vi "Ethernet Packet Counter for Testing.vi"() -> ()   [LabVIEW 2025]
uses:
  <vilib>/xnet/xnet.llb/XNET Frame Type Ethernet.ctl
  <vilib>/xnet/xnet.llb/XNET Create Session (Frame Output Stream).vi
  <vilib>/xnet/xnet.llb/XNET Write (Frame Ethernet).vi
  Automotive Ethernet Bus Monitor/Automotive Ethernet Bus Monitor.lvclass
panel:
  out "error out":errorcluster
  in  "destination MAC address":cluster{u8, u8, u8, u8, u8, u8}={255, 255, 255, 255, 255, 255} {"?" format="%.0x"; "?" format="%.0x"; "?" format="%.0x"; "?" format="%.0x"; "?" format="%.0x"; "?" format="%.0x"}
  in  "Has VLAN Tag 2":bool=TRUE
  in  "VID 2":u16=2
  in  "priority":u8=3
  in  "Stop":bool
  out "Number of Frames Sent":i32
  in  "Ethertype":u16=1 format="%.0x"
  in  "Interface":refnum<k21>="ENET1"
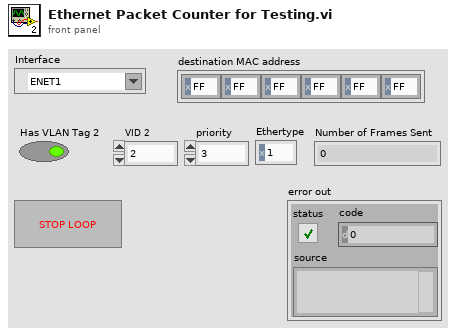
[diagram p1: front panel]
types:
  T1 = typedef "XNET Frame Type Ethernet.ctl" = u16
  T2 = cluster{"local timestamp":timestamp, "network timestamp":timestamp, "frame data":u8[], "fcs":u32, "type":T1, "network synced?":bool, "receive?":bool, "transmit?":bool, "error?":bool}
  T3 = cluster{"destination MAC address":cluster{u8, u8, u8, u8, u8, u8}, "source MAC address":cluster{u8, u8, u8, u8, u8, u8}, "Has VLAN Tag":bool, "VLAN Tag":cluster{"TPID":u16, "priority":u8, "DEI":bool, "VID":u16}, "Ethertype":u16}
  T4 = cluster{"TPID":u16, "priority":u8, "DEI":bool, "VID":u16}
  T5 = cluster{"local timestamp":timestamp, "network timestamp":timestamp, "frame data":u8[], "fcs":u32, "type":T1, "network synced?":bool, "receive?":bool, "transmit?":bool, "error?":bool}[]
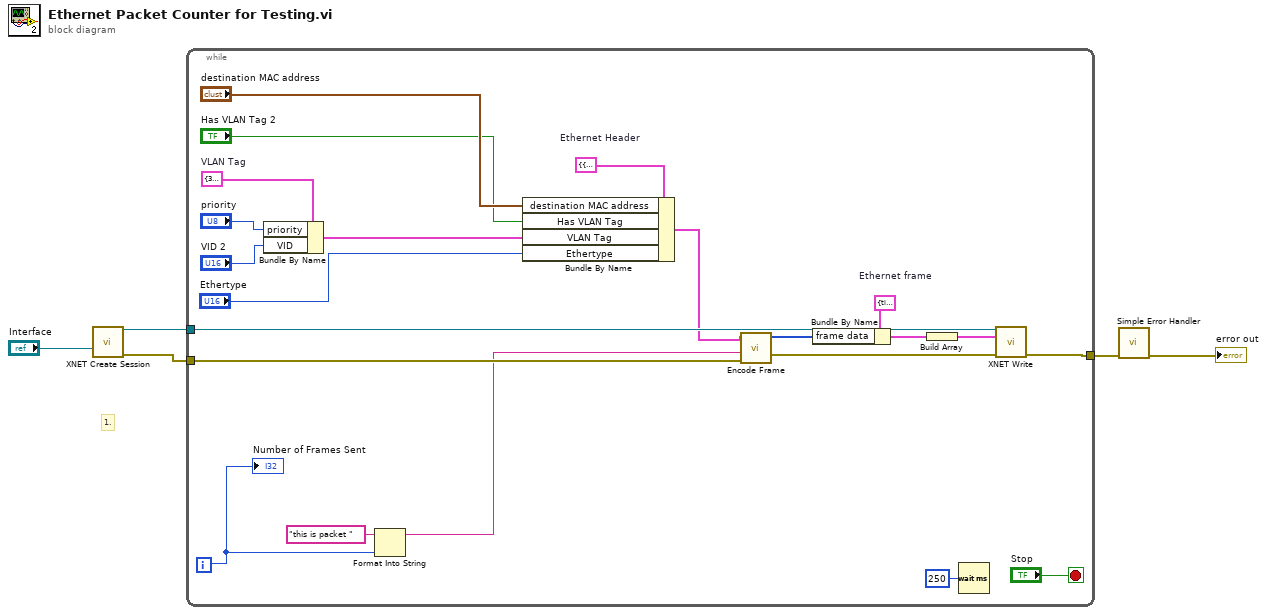
[diagram p0: block diagram]
diagram:
  # "1."
  n1 = call-poly <vilib>:"XNET Create Session.vi"("interface"="Interface") -> ("session out"=w4:refnum<k21>, "error out"=w2:errorcluster)  [unwired: 13 in]
  n2 = while {
    tunnel: w4 -> [w27]
    tunnel: [w24] -> w3
    tunnel: w2 -> [w10]
    i -> [w8]
    stop <- "Stop" stop-if-true
    w18 = T2 {"local timestamp"=timestamp(0 s since 1904-01-01), "network timestamp"=timestamp(0 s since 1904-01-01), "frame data"=[], "fcs"=0, "type"=0, "network synced?"=FALSE, "receive?"=FALSE, "transmit?"=FALSE, "error?"=FALSE}  # Ethernet frame
    w23 = T3 {"destination MAC address"={0, 0, 0, 0, 0, 0}, "source MAC address"={0, 0, 0, 0, 0, 0}, "Has VLAN Tag"=FALSE, "VLAN Tag"={"TPID"=33024, "priority"=0, "DEI"=FALSE, "VID"=0}, "Ethertype"=0}  # Ethernet Header
    w22 = T4 {"TPID"=33024, "priority"=0, "DEI"=FALSE, "VID"=0}  # VLAN Tag
    n3 = Bundle By Name(cluster=w22, "priority"="priority", "VID"="VID 2") -> (w21:T4)
    n4 = Format Into String(initial string="this is packet ", w8) -> (resulting string=w7:string)  [unwired: 2 in, 1 out]
    n5 = Bundle By Name(cluster=w23, "destination MAC address"="destination MAC address", "Has VLAN Tag"="Has VLAN Tag 2", "VLAN Tag"=w21, "Ethertype"="Ethertype") -> (w13:T3)
    n6 = call "Encode Frame.vi"("error in (no error)"=w10, "payload"=w7, "Ethernet Header"=w13) -> ("error out"=w11:errorcluster, "frame data"=w12:u8[])  [unwired: 7 in]
    n7 = Bundle By Name(cluster=w18, "frame data"=w12) -> (w17:T2)
    n8 = Build Array(w17) -> (w16:T5)
    n9 = Wait (ms)(milliseconds to wait=u32 250) -> ()  [unwired: 1 out]
    n10 = call-poly <vilib>:"XNET Write.vi"("session in"=w27, "data"=w16, "error in (no error)"=w11) -> ("error out"=w24:errorcluster)  [unwired: 11 in, 1 out]
    "Number of Frames Sent" <- w8
  }
  n11 = call <vilib>:"Simple Error Handler.vi"("error in (no error)"=w3) -> ("error out"=→"error out":errorcluster)  [unwired: 4 in, 4 out]
